vi "WaitForConnection.vi"(8 "error in (no error)":errorcluster, 11 "TcpServer in":refnum<class "TcpServer.lvclass">) -> (0 "error out":errorcluster, 2 "Connection":refnum<class "Connection.lvclass">, 3 "TcpServer out":refnum<class "TcpServer.lvclass">)   [LabVIEW 2021, in "TcpServer.lvlib" / "TcpServer.lvclass"]
uses:
  TcpServer.lvclass
  TcpServer.lvclass/TcpServer.ctl
  Connection/Connection.lvclass
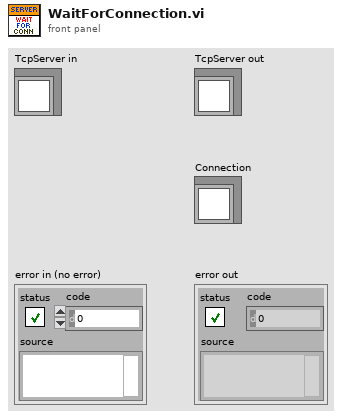
[diagram p1: front panel]
types:
  T1 = enum16{"Standard", "Buffered", "CRLF", "Immediate"}
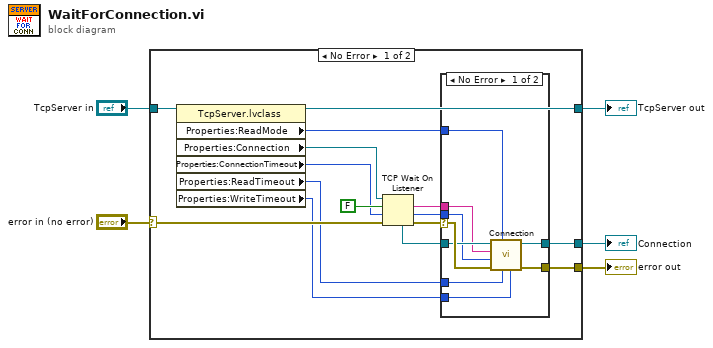
[diagram p0: block diagram]
diagram:
  n1 = case shown="No Error" "error in (no error)" {
    selector: "error in (no error)" -> [w19 w32]
    tunnel: [w16 w32] -> w4
    tunnel: [w11 w31] -> w2
    tunnel: "TcpServer in" -> [w20 w31]
    tunnel: [w12 _] -> w1
    frame No Error {
      n2 = property class="TcpServer.lvclass"(reference=w20) -> (reference out=w11:refnum<class "TcpServer.lvclass">, "Properties:ReadMode"=w10:T1, "Properties:Connection"=w9:refnum<k5>, "Properties:ConnectionTimeout"=w8:i32, "Properties:ReadTimeout"=w7:i32, "Properties:WriteTimeout"=w6:i32)  [unwired: 1 in, 1 out]
      n3 = TCP Wait On Listener(8:w19, 9:w8, 10:FALSE ("resolve remote address (T)"), 11:w9) -> (0:w17:errorcluster, 1:w14:u16, 2:w15:string, 4:w13:refnum<k5>)  [unwired: 1 out]
      n4 = case shown="No Error" w17 {
        selector: w17 -> [w29 w30]
        tunnel: [w26 w30] -> w16
        tunnel: w15 -> [w23 _]
        tunnel: w14 -> [w24 _]
        tunnel: w13 -> [w25 _]
        tunnel: [w28 _] -> w12
        tunnel: w10 -> [w27 _]
        tunnel: w7 -> [w22 _]
        tunnel: w6 -> [w21 _]
        frame No Error {
          n5 = call "Connection.vi"("WriteTimeout [ms] (5000)"=w21, "ReadTimeout [ms] (5000)"=w22, "ReadMode (Standard)"=w27, "error in (no error)"=w29, "Port"=w24, "Address"=w23, "Connection"=w25) -> ("error out"=w26:errorcluster, "Connection"=w28:refnum<class "Connection.lvclass">)  [unwired: 3 in]
        }
        frame Error {
        }
      }
    }
    frame Error {
    }
  }
  "error out" <- w4
  "TcpServer out" <- w2
  "Connection" <- w1
